vi "Overall_system_A2-125khz.vi"() -> ()   [LabVIEW 2019]
doc: "This VI is th overall VI that can read the weight, rfid and camera (and save the data into a csv file). When certain threshold are met it can also send a telegram message at the end."
uses:
  dependencies/notification/Telegram-Bot-master (1)/Telegram-Bot-master/Telegram/Methods/TypeDefs/SendMessageType.ctl
panel:
  out "Rfid 2":string
  in  "RFID VISA resource name 2":refnum<visa-resource-name>="COM18"
  out "Rfid":string
  in  "RFID VISA resource name":refnum<visa-resource-name>="COM5"
  in  "start condition (debug)":bool
  out "Weight":string
  in  "delay before read (ms)":u32=500
  in  "Weight VISA resource name":refnum<visa-resource-name>="COM1"
  in  "Start camera (debug)":bool
  out "Health Monitoring in Progress":bool
  in  "Bird is underfeeding (debug)":bool
  out "Current image":T1(plugin-control)
  in  "Camera Name":refnum<k21>="cam0" caption="IMAQdx Session"
  # "Intelligent Health Monitoring System"
  # "grams"
  # "Weight detection settings:"
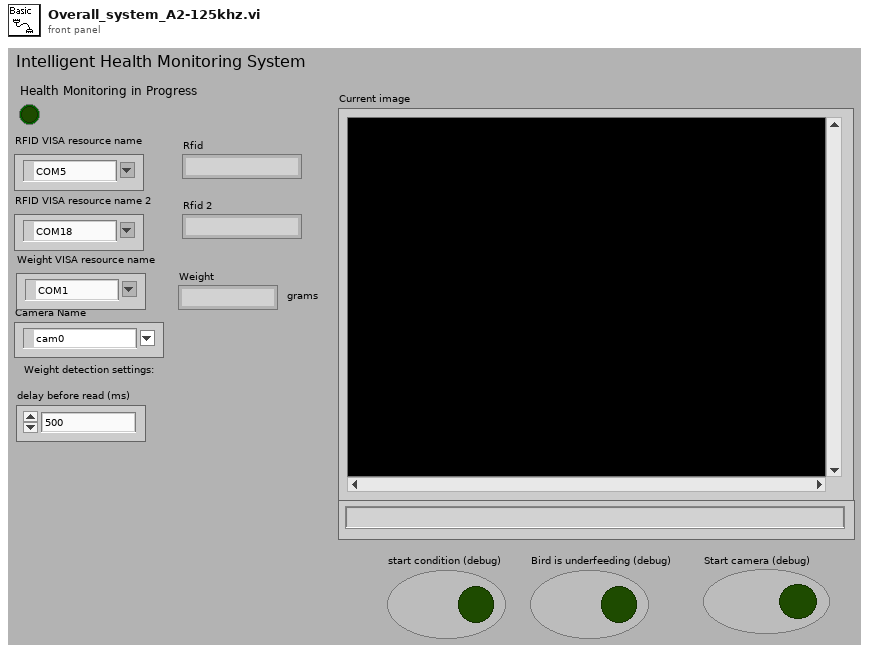
[diagram p1: front panel]
types:
  T1 = typedef "IMAQ Image.ctl" = refnum<image>
  T2 = typedef "SendMessageType.ctl" = enum16{"Text", "ReplyKeyboardMarkup", "ReplyKeyboardRemove"}
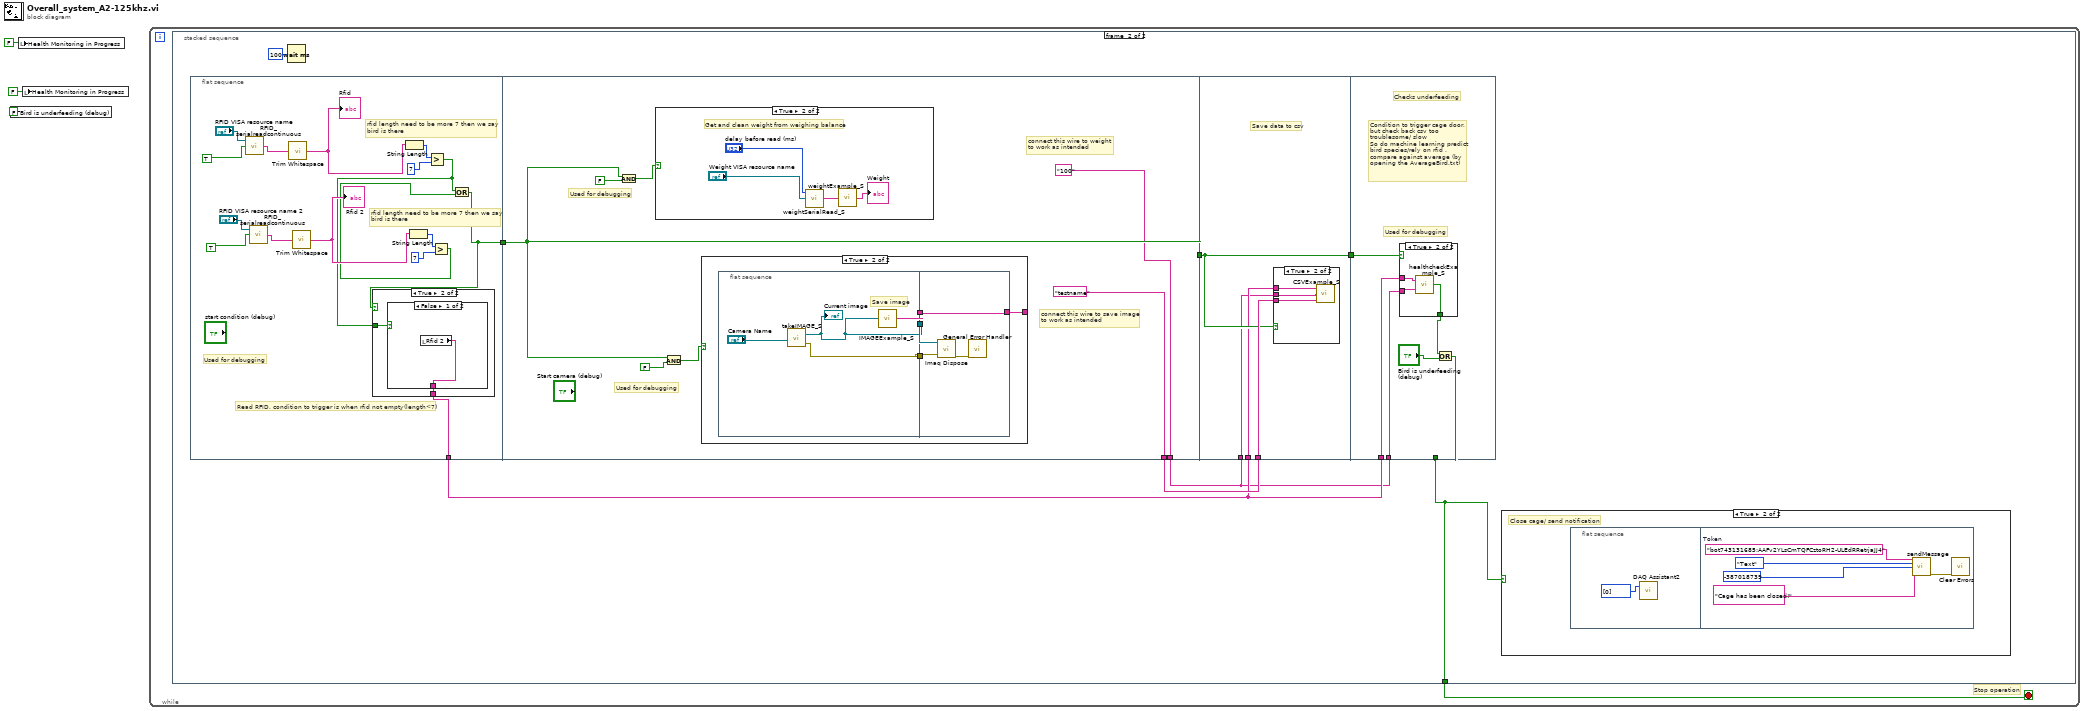
[diagram p0: block diagram]
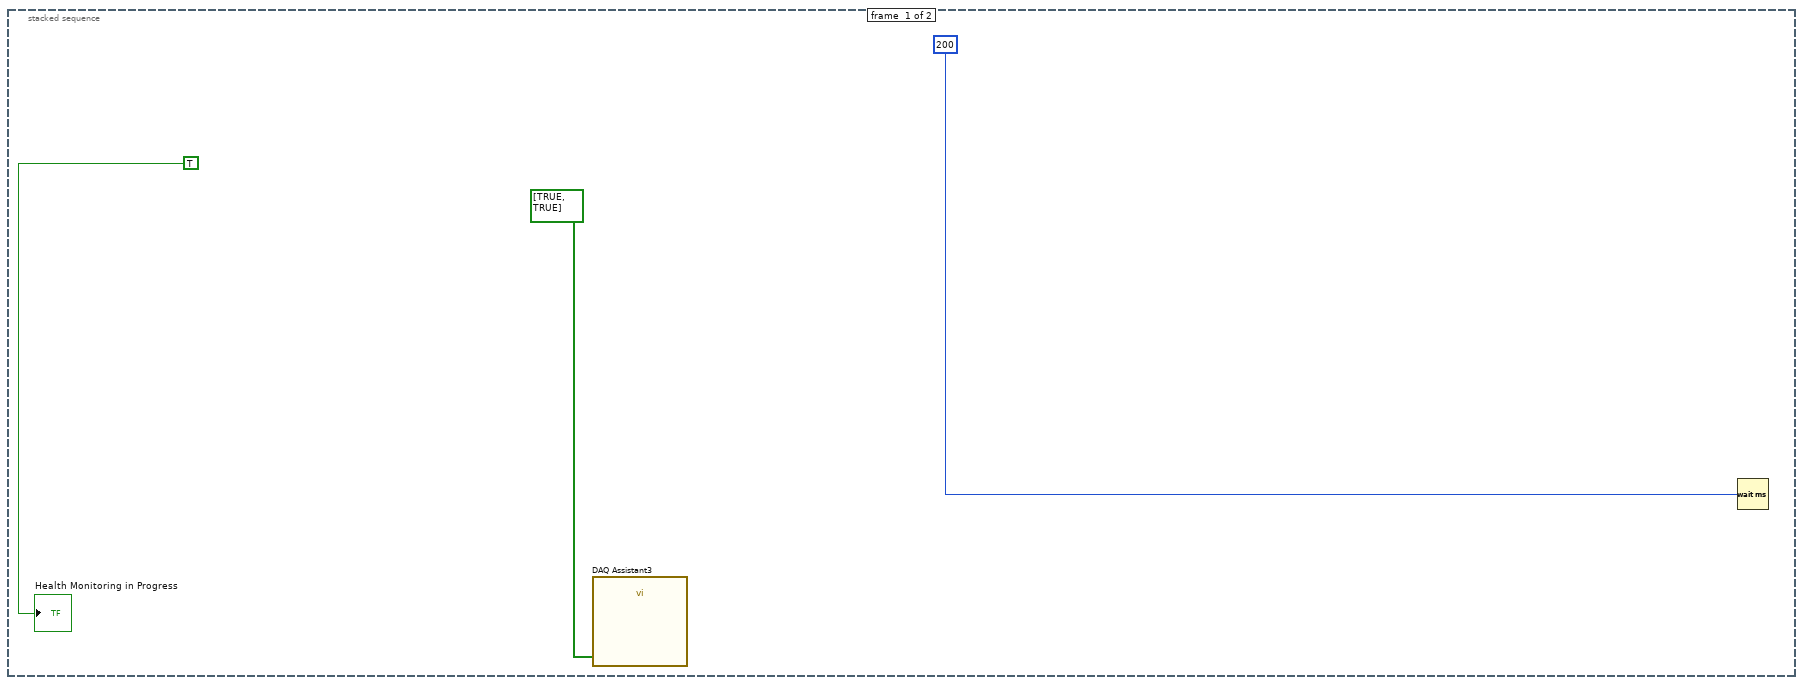
[diagram p2: hidden frame]
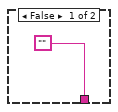
[diagram p3: hidden frame]
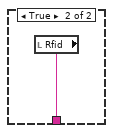
[diagram p4: hidden frame]
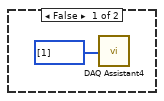
[diagram p6: hidden frame]
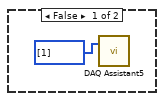
[diagram p9: hidden frame]
diagram:
  n1 = local write "Bird is underfeeding (debug)"(FALSE ("Bird is underfeeding")) -> ()
  n2 = local write "Health Monitoring in Progress"(FALSE ("Health Monitoring in Progress")) -> ()
  n3 = local write "Health Monitoring in Progress"(FALSE ("Health Monitoring in Progress")) -> ()
  n4 = while {
    stop <- w4 stop-if-true
    # "Stop operation"
    n5 = stacked-sequence {
      tunnel: [_ w14] -> w4
      frame #0 {
        n6 = call "DAQ Assistant3"("data"=bool[] [TRUE, TRUE]) -> ()  [unwired: 17 in, 2 out]
        n7 = Wait (ms)(milliseconds to wait=u32 200) -> ()  [unwired: 1 out]
        "Health Monitoring in Progress" <- TRUE ("Health Monitoring in Progress")
      }
      frame #1 {
        n8 = flat-sequence {
          tunnel: [w16] -> w9
          tunnel: [w18] -> w13
          tunnel: ["100"] -> w8
          tunnel: ["testname"] -> w10
          tunnel: w13 -> [w39]
          tunnel: [w39] -> w12
          tunnel: w12 -> [w63]
          tunnel: [w63] -> w11
          tunnel: w10 -> [w64]
          tunnel: w9 -> [w62]
          tunnel: w8 -> [w61]
          tunnel: [w70] -> w14
          tunnel: w9 -> [w69]
          tunnel: w11 -> [w73]
          tunnel: w8 -> [w68]
          frame #0 {
            # "rfid length need to be more 7 then we say \nbird is there"
            # "Used for debugging"
            # "rfid length need to be more 7 then we say \nbird is there"
            # "Read RFID, condition to trigger is when rfid not empty(length<7)"
            n9 = call "RFID_serialreadcontinuous.vi"("Read 2"=TRUE, "VISA resource name"="RFID VISA resource name") -> ("Response 2"=w28:string)  [unwired: 1 in]
            n10 = call "RFID_serialreadcontinuous.vi"("Read 2"=TRUE, "VISA resource name"="RFID VISA resource name 2") -> ("Response 2"=w23:string)  [unwired: 1 in]
            n11 = call <vilib>:"Trim Whitespace.vi"("string"=w28) -> ("trimmed string"=w29:string)  [unwired: 1 in]
            "Rfid" <- w29
            n12 = call <vilib>:"Trim Whitespace.vi"("string"=w23) -> ("trimmed string"=w24:string)  [unwired: 1 in]
            "Rfid 2" <- w24
            n13 = String Length(string=w29) -> (length=w31:i32)
            n14 = String Length(string=w24) -> (length=w25:i32)
            n15 = Greater?(x=w31, y=7) -> (0:w17:bool)
            n16 = Greater?(x=w25, y=7) -> (0:w19:bool)
            n17 = Or(x=w17, y=w19) -> (x .or. y?=w18:bool)
            n18 = case shown="True" w18 {
              tunnel: w17 -> [_ w34]
              tunnel: ["" w33] -> w16
              frame False {
              }
              frame True {
                n19 = case shown="False" w34 {
                  tunnel: [w35 w36] -> w33
                  frame False {
                    n20 = local read "Rfid 2"() -> (w35:string)
                  }
                  frame True {
                    n21 = local read "Rfid"() -> (w36:string)
                  }
                }
              }
            }
          }
          frame #1 {
            # "connect this wire to save image \nto work as intended"
            # "connect this wire to weight \nto work as intended"
            # "Used for debugging"
            # "Used for debugging"
            n22 = And(x=w39, y=FALSE) -> (x .and. y?=w38:bool)
            n23 = case shown="True" w38 {
              frame False {
                n24 = call "DAQ Assistant4"("data"=u32[] [1]) -> ()  [unwired: 17 in, 2 out]
              }
              frame True {
                # "Get and clean weight from weighing balance"
                n25 = call "weightSerialRead_S.vi"("Weight VISA resource name"="Weight VISA resource name", "delay before read (ms)"="delay before read (ms)") -> ("String"=w60:string)  [unwired: 1 in]
                n26 = call "weightExample_S.vi"("weight"=w60) -> ("String"=→"Weight":string)
              }
            }
            n27 = And(x=w39, y=FALSE) -> (x .and. y?=w42:bool)
            n28 = case shown="True" w42 {
              tunnel: [_ w45] -> _
              frame False {
              }
              frame True {
                n29 = flat-sequence {
                  tunnel: [w49] -> w47
                  tunnel: [w48] -> w46
                  tunnel: [w51] -> w44
                  tunnel: w47 -> [w55]
                  tunnel: w46 -> [w53]
                  tunnel: [w52] -> w45
                  tunnel: w44 -> [w52]
                  frame #0 {
                    # "Save image"
                    n30 = call "takeIMAGE_S.vi"("Camera Name"="Camera Name") -> ("Current image"=w48:T1, "error in (no error)"=w49:errorcluster)
                    "Current image" <- w48
                    n31 = call "IMAGEExample_S.vi"("Image"=w48) -> ("String"=w51:string)
                  }
                  frame #1 {
                    n32 = call "Imaq Dispose"("Image"=w53, "error in (no error)"=w55) -> ("error out"=w54:errorcluster)  [unwired: 4 in]
                    n33 = call <vilib>:"General Error Handler.vi"("error in (no error)"=w54) -> ()  [unwired: 2 in, 13 out]
                  }
                }
              }
            }
          }
          frame #2 {
            # "Save data to csv"
            n34 = case shown="True" w63 {
              tunnel: w64 -> [_ w65]
              tunnel: w61 -> [_ w66]
              tunnel: w62 -> [_ w67]
              frame False {
              }
              frame True {
                n35 = call "CSVExample_S.vi"("imageId"=w65, "weight"=w66, "rfid"=w67) -> ()
              }
            }
          }
          frame #3 {
            # "Used for debugging"
            # "Condition to trigger cage door,\nbut check back csv too troublesome/ slow\nSo do machine learning predict bird species/rely on rfid , compare against average (by opening the AverageBird.txt)"
            # "Checks underfeeding"
            n36 = case shown="True" w73 {
              tunnel: [_ w74] -> w72
              tunnel: w69 -> [_ w75]
              tunnel: w68 -> [_ w76]
              frame False {
              }
              frame True {
                n37 = call "healthcheckExample_S.vi"("weight"=w76, "rfid"=w75) -> ("Boolean"=w74:bool)
              }
            }
            n38 = Or(x=w72, y="Bird is underfeeding (debug)") -> (x .or. y?=w70:bool)
          }
        }
        n39 = Wait (ms)(milliseconds to wait=u32 100) -> ()  [unwired: 1 out]
        n40 = case shown="True" w14 {
          frame False {
            n41 = call "DAQ Assistant5"("data"=u32[] [1]) -> ()  [unwired: 17 in, 2 out]
          }
          frame True {
            # "Close cage/ send notification"
            n42 = flat-sequence {
              frame #0 {
                n43 = call "DAQ Assistant2"("data"=u32[] [0]) -> ()  [unwired: 17 in, 2 out]
              }
              frame #1 {
                w82 = "bot743131685:AAFv2YLsCmTQFCztoRH2-ULEdRRetrjaJJ4"  # Token
                n44 = call "sendMessage.vi"("Token"=w82, "MsgType"=SendMessageType."Text", "ChatId"=i64 -387018739, "Text"="Cage has been closed!") -> ("error out"=w83:errorcluster)  [unwired: 11 in]
                n45 = call <vilib>:"Clear Errors.vi"("error in (no error)"=w83) -> ()  [unwired: 5 in, 2 out]
              }
            }
          }
        }
      }
    }
  }
